vi "Write Custom SCP Commands List Property.vi"(6 "Remove 1st Column? (T)":bool=TRUE, 8 "error in (no error)":errorcluster, 10 "Custom SCP Commands List":string[][](array[string]), 11 "Node Ptr":T1 format="%.0x") -> (0 "error out":errorcluster, 3 "Item Ref out":T1 format="%.0x")   [LabVIEW 2018, in "Vires VTD System Explorer.lvlib"]
doc: "Removes first column and writes 2D array of strings to CD Item Property"
uses:
  Vires VTD System Explorer.lvlib
  <vilib>/NI Veristand/Custom Device API/Custom Device Item Ref.ctl
  Shared/Constants.vi
  <vilib>/NI Veristand/Custom Device API/Set Item Property (Variant).vi
  Shared/Vires VTD Shared.lvlib
  <vilib>/NI Veristand/Custom Device API/Custom Device API.lvlib
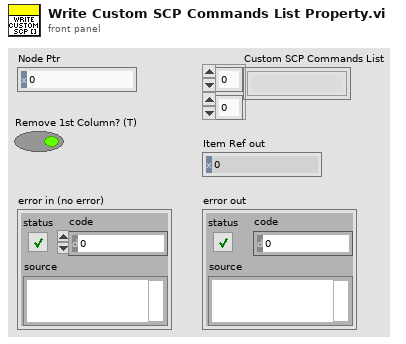
[diagram p1: front panel]
types:
  T1 = typedef "Custom Device API.lvlib/Custom Device Item Ref.ctl" = u64
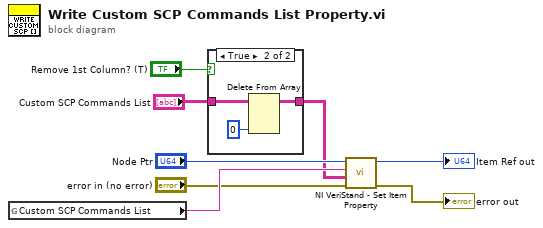
[diagram p0: block diagram]
diagram:
  n1 = global read "Constants.vi" "Custom SCP Commands List"() -> (w8:string)
  n2 = case shown="True" "Remove 1st Column? (T)" {
    tunnel: "Custom SCP Commands List" -> [w9 w12]
    tunnel: [w9 w10] -> w2
    frame False {
    }
    frame True {
      n3 = Delete From Array(array=w12, index (col)=0 ("disabled index (col)")) -> (array with subset deleted=w10:string[][])  [unwired: 2 in, 1 out]
    }
  }
  n4 = call-poly <vilib>:"NI VeriStand - Set Item Property.vi"("error in (no error)"="error in (no error)", "Value"=w2, "Property Name"=w8, "Item Ref in"="Node Ptr") -> ("error out"=→"error out":errorcluster, "Item Ref out"=→"Item Ref out":T1)  [unwired: 5 in, 1 out]
